vi "Solve2.vi"(8 "Error In":errorcluster, 11 "object in":refnum<class "2024_6.lvclass">) -> (0 "Error Out":errorcluster, 2 "Result":u64, 3 "object out":refnum<class "2024_6.lvclass">)   [LabVIEW 2023, in "2024_6.lvclass"]
uses:
  2024_6.lvclass
  2024_6.lvclass/2024_6.ctl
  <vilib>/Utility/miscctls.llb/LVMapReplaceAction.ctl
  03272fe1-dcf6-4c00-ac4b-605355b719d0.vi
panel:
  out "Array":cluster{"X":i32, "Y":i32}[](array[cluster])
  out "Current Direction":enum16{"Up", "Right", "Down", "Left"}(ring)
  out "map":u32[][](array[colorbox])
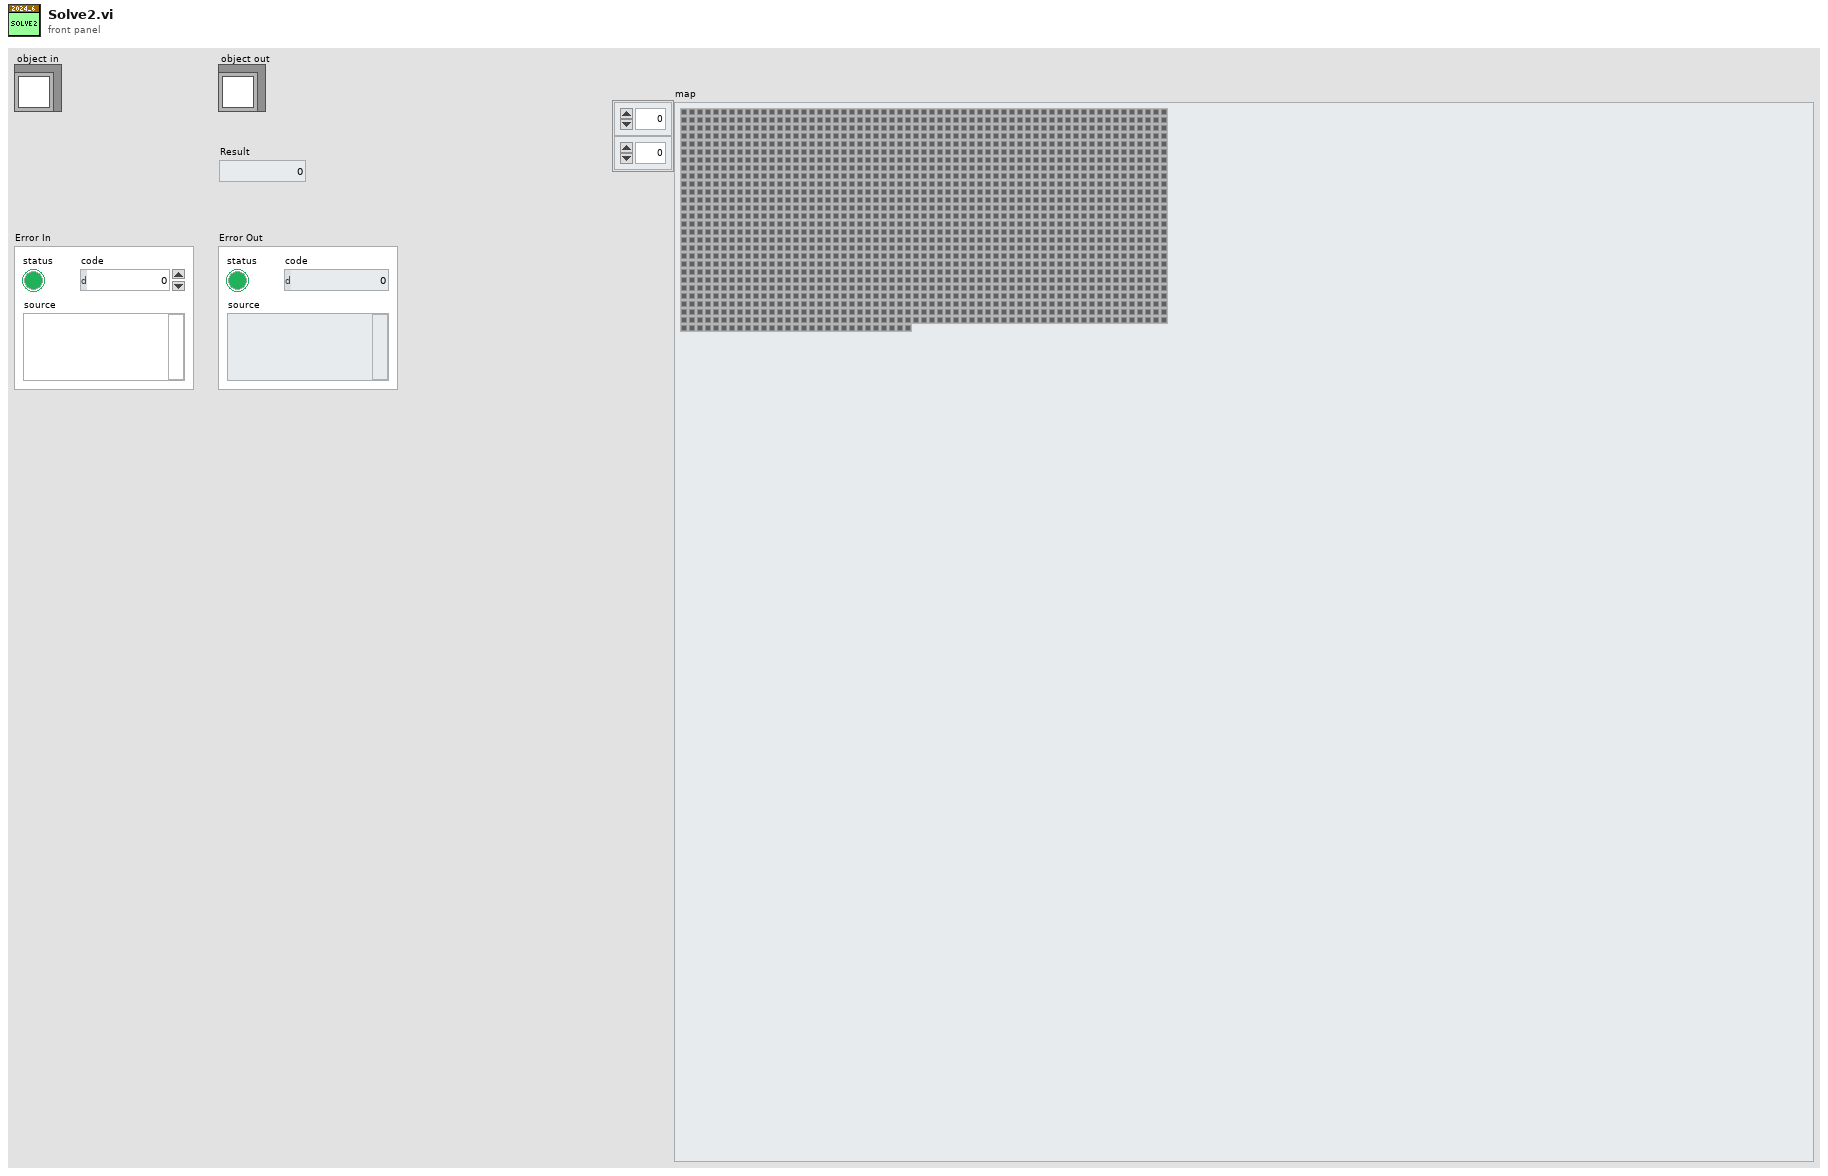
[diagram p1: front panel]
types:
  T1 = map{cluster{"X":i32, "Y":i32}, set{enum16{"Up", "Right", "Down", "Left"}}}
  T2 = typedef "LVMapReplaceAction.ctl" = enum32{"Modify Entry only if found", "Add or Modify Entry", "Delete Entry"}
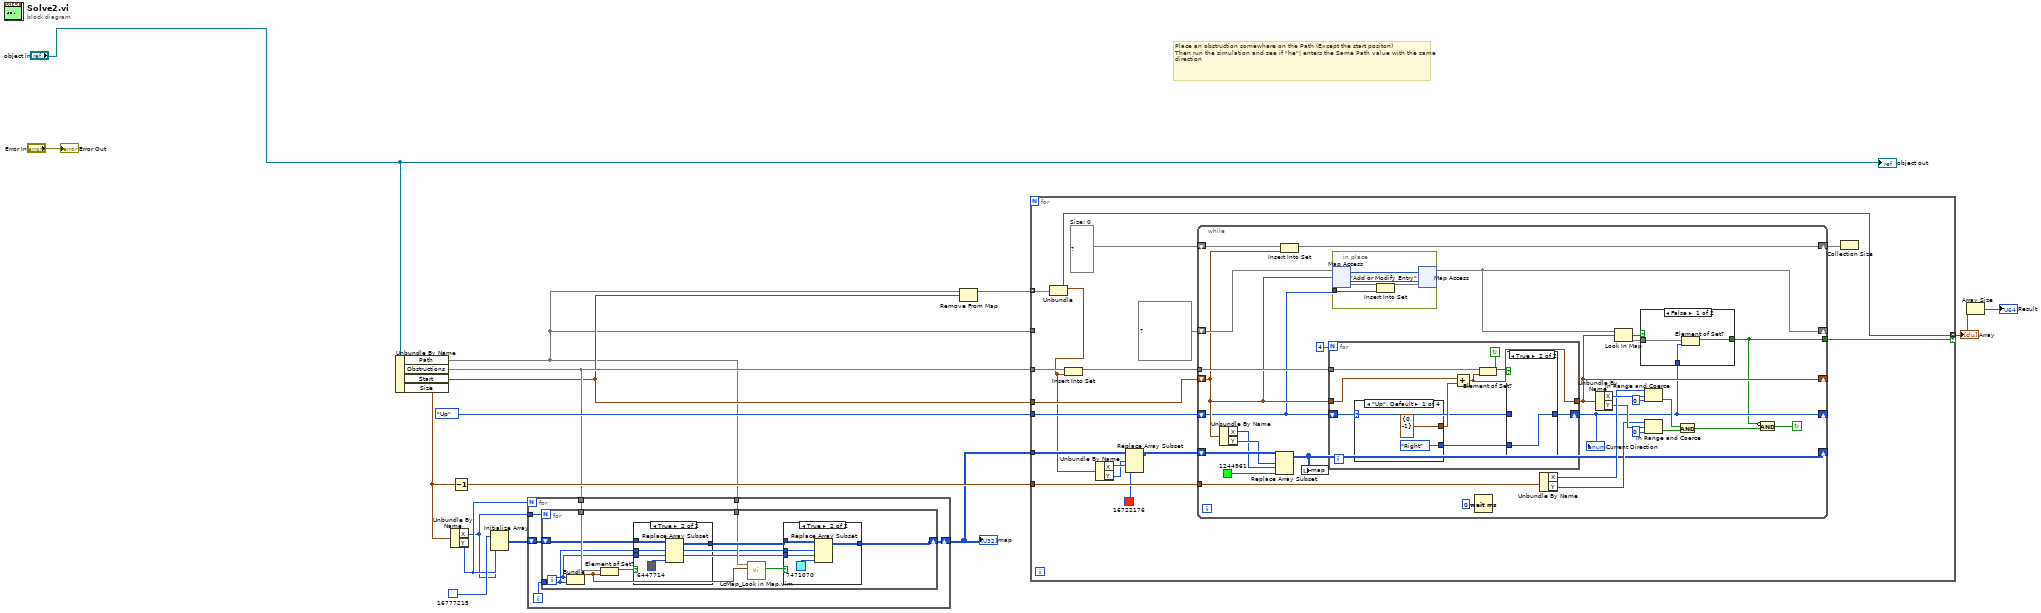
[diagram p0: block diagram]
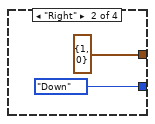
[diagram p4: hidden frame]
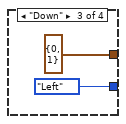
[diagram p5: hidden frame]
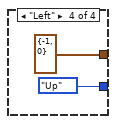
[diagram p6: hidden frame]
diagram:
  # "Place an obstruction somewhere on the Path (Except the start positon)\nThen run the simulation and see if \"he\"| enters the Same Path value with the same direction"
  n1 = Unbundle By Name("object in") -> ("Path"=w1:T1, "Obstructions"=w10:set{cluster{"X":i32, "Y":i32}}, "Start"=w5:cluster{"X":i32, "Y":i32}, "Size"=w13:cluster{"X":i32, "Y":i32})
  n2 = Unbundle By Name(w13) -> ("X"=w8:i32, "Y"=w9:i32)
  n3 = Decrement(x=w13) -> (x-1=w14:cluster{"X":i32, "Y":i32})
  n4 = Initialize Array(u32 16777215, w9, w8) -> (w11:u32[][])
  n5 = for {
    N: w9 -> [_]
    tunnel: w10 -> [w20]
    shift-right: [w18] -> w7
    shift-left: w11 -> [w22]
    tunnel: w8 -> [w19]
    tunnel: w1 -> [w17]
    i -> [w21]
    n6 = for {
      N: w19 -> [_]
      tunnel: w21 -> [w24]
      tunnel: w20 -> [w32]
      shift-right: [w28] -> w18
      shift-left: w22 -> [w30]
      tunnel: w17 -> [w27]
      i -> [w23]
      n7 = Bundle(w23, w24) -> (w26:cluster{i32, i32})  [unwired: 1 in]
      n8 = Element of Set?(10:w26, 11:w32) -> (3:w31:bool)
      n9 = case shown="True" w31 {
        tunnel: w30 -> [w39 w44]
        tunnel: w24 -> [_ w43]
        tunnel: w23 -> [_ w42]
        tunnel: [w39 w40] -> w29
        frame False {
        }
        frame True {
          n10 = Replace Array Subset(array=w44, new element=u32 6447714, index (row)=w43, index (col)=w42) -> (w40:u32[][])
        }
      }
      n11 = call "LcMap_Look in Map.vim"("key"=w26, "map"=w27) -> ("key found?"=w25:bool)  [unwired: 8 in, 1 out]
      n12 = case shown="True" w25 {
        tunnel: w29 -> [w33 w38]
        tunnel: w24 -> [_ w37]
        tunnel: w23 -> [_ w36]
        tunnel: [w33 w34] -> w28
        frame False {
        }
        frame True {
          n13 = Replace Array Subset(array=w38, new element=u32 7471070, index (row)=w37, index (col)=w36) -> (w34:u32[][])
        }
      }
    }
  }
  "map" <- w7
  n14 = Remove From Map(10:w5, 11:w1) -> (3:w4:T1)  [unwired: 2 out]
  n15 = for {
    tunnel: enum16{"Up", "Right", "Down", "Left"}."Up" -> [w60]
    tunnel: w14 -> [w58]
    tunnel: w10 -> [w56]
    tunnel: w7 -> [w51]
    tunnel: w1 -> [_]
    tunnel: w5 -> [w55]
    tunnel: w4 -> [w54] mode=indexing
    tunnel: [w49] -> w3 mode=indexing if=w53
    w59 = set{cluster{"X":i32, "Y":i32}} {}  # Size: 0
    n16 = Unbundle(w54) -> ("Path"=w49:cluster{"X":i32, "Y":i32})  [unwired: 1 out]
    n17 = Insert Into Set(10:w49, 11:w56) -> (3:w52:set{cluster{"X":i32, "Y":i32}})  [unwired: 1 out]
    n18 = Unbundle By Name(w49) -> ("X"=w48:i32, "Y"=w47:i32)
    n19 = Replace Array Subset(array=w51, new element=u32 16722176, index (row)=w47, index (col)=w48) -> (w50:u32[][])
    n20 = while {
      shift-right: [w70] -> _
      shift-left: w55 -> [w63]
      shift-right: [w67] -> _
      shift-left: w60 -> [w62]
      shift-right: [w77] -> w57
      shift-left: w59 -> [w90]
      tunnel: w58 -> [w87]
      tunnel: w52 -> [w82]
      shift-right: [w72] -> _
      shift-left: w50 -> [w76]
      tunnel: [w65] -> w53
      shift-right: [w61] -> _
      shift-left: T1 {} ("Path") -> [w64]
      stop <- w66 continue-if-true
      n21 = Unbundle By Name(w63) -> ("X"=w74:i32, "Y"=w75:i32)
      n22 = Replace Array Subset(array=w76, new element=u32 1244961, index (row)=w75, index (col)=w74) -> (w72:u32[][])
      n23 = Insert Into Set(10:w63, 11:w90) -> (3:w77:set{cluster{"X":i32, "Y":i32}})  [unwired: 1 out]
      n24 = local write "map"(w72) -> ()
      n25 = for {
        N: 4 -> [_]
        tunnel: w82 -> [w103]
        shift-right: [w99] -> w67
        shift-left: w62 -> [w100]
        tunnel: w63 -> [w105]
        tunnel: [w102] -> w70
        stop <- w101 continue-if-true
        n26 = case shown="\"Up\", Default" w100 {
          tunnel: [cluster{"X":i32, "Y":i32} {"X"=0, "Y"=-1} ("y") cluster{"X":i32, "Y":i32} {"X"=1, "Y"=0} ("y") cluster{"X":i32, "Y":i32} {"X"=0, "Y"=1} ("y") cluster{"X":i32, "Y":i32} {"X"=-1, "Y"=0} ("y")] -> w104
          tunnel: [enum16{"Up", "Right", "Down", "Left"}."Right" enum16{"Up", "Right", "Down", "Left"}."Down" enum16{"Up", "Right", "Down", "Left"}."Left" enum16{"Up", "Right", "Down", "Left"}."Up"] -> w98
          frame "Up", Default {
          }
          frame "Right" {
          }
          frame "Down" {
          }
          frame "Left" {
          }
        }
        n27 = Add(x=w105, y=w104) -> (x+y=w102:cluster{"X":i32, "Y":i32})
        n28 = Element of Set?(10:w102, 11:w103) -> (3:w101:bool)
        n29 = case shown="True" w101 {
          tunnel: w100 -> [w106 _]
          tunnel: [w106 w107] -> w99
          tunnel: w98 -> [_ w107]
          frame False {
          }
          frame True {
          }
        }
      }
      "Current Direction" <- w67
      n30 = in-place {
        in-place-border: w62 -> [w93]
        n31 = in-place-map #1(w64, w63) -> (w94:set{enum16{"Up", "Right", "Down", "Left"}})  [unwired: 1 in, 1 out]
        n32 = Insert Into Set(10:w93, 11:w94) -> (3:w92:set{enum16{"Up", "Right", "Down", "Left"}})  [unwired: 1 out]
        n33 = in-place-map #1(w92, LVMapReplaceAction."Add or Modify Entry" ("action")) -> (w61:T1)  [unwired: 2 out]
      }
      n34 = Wait (ms)(milliseconds to wait=u32 0) -> ()  [unwired: 1 out]
      n35 = Unbundle By Name(w87) -> ("X"=w86:i32, "Y"=w83:i32)
      n36 = Unbundle By Name(w70) -> ("X"=w89:i32, "Y"=w84:i32)
      n37 = Look In Map(map=w61, key=w70) -> (key not found?=w69:bool, value=w68:set{enum16{"Up", "Right", "Down", "Left"}})  [unwired: 1 in]
      n38 = case shown="False" w69 {
        tunnel: w68 -> [w97 _]
        tunnel: w67 -> [w96 _]
        tunnel: [w95 _] -> w65
        frame False {
          n39 = Element of Set?(10:w96, 11:w97) -> (3:w95:bool)
        }
        frame True {
        }
      }
      n40 = In Range and Coerce(upper limit=w86, x=w89, lower limit=0) -> (In Range?=w79:bool)  [unwired: 1 out]
      n41 = In Range and Coerce(upper limit=w83, x=w84, lower limit=0) -> (In Range?=w80:bool)  [unwired: 1 out]
      n42 = And(x=w79, y=w80) -> (x .and. y?=w78:bool)
      n43 = Compound Arithmetic op=AND(invert w65, w78) -> (w66:bool)
    }
    n44 = Collection Size(1:w57) -> ()  [unwired: 1 out]
  }
  "Array" <- w3
  n45 = Array Size(array=w3) -> (size(s)=→"Result":i32)
  "Error Out" <- "Error In"
  "object out" <- "object in"
